vi "my_1D_sample-tip-convolution.vi"() -> ()   [LabVIEW 2017]
panel:
  out "Waveform Graph":dbl[][](graph)
  in  "stop":bool
  in  "scanning speed":u32(slide)=66 scale=1.0..1000.0
  in  "Angle":dbl=1.0 min=1.0 max=89.0 format="%.2f"
  in  "Radius":dbl min=-0.0 max=1000.0 format="%.2f"
  in  "Length":i32=1000
  in  "Period":dbl=310.0 format="%.2f"
  in  "Height":dbl=120.0 format="%.2f"
  in  "Width":dbl=140.0 format="%.2f"
  in  "Slope":dbl=1.0 format="%.2f"
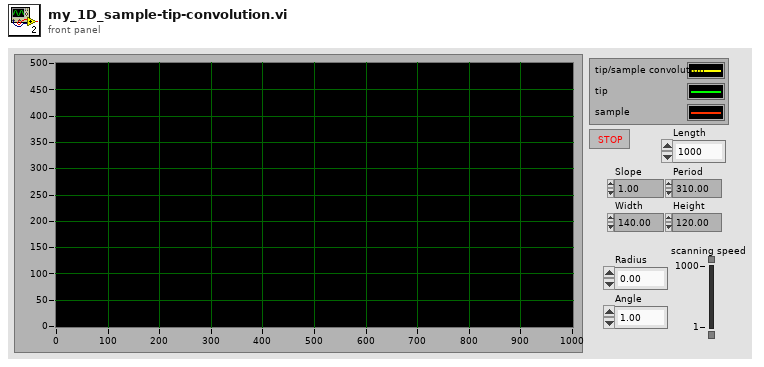
[diagram p1: front panel]
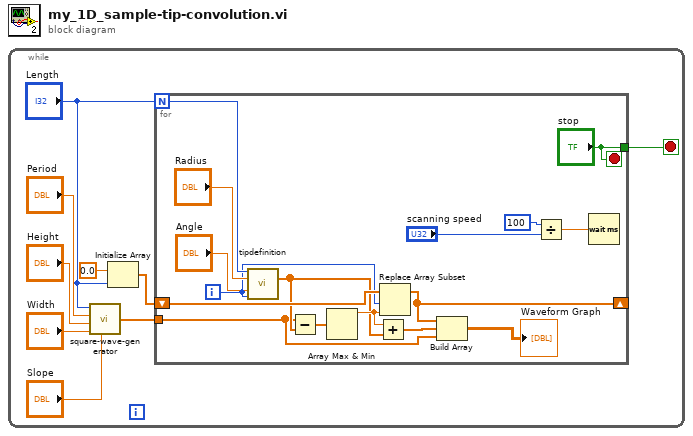
[diagram p0: block diagram]
diagram:
  n1 = while {
    stop <- w1 stop-if-true
    n2 = call "square-wave-generator.vi"("Slope"="Slope", "Width"="Width", "Height"="Height", "Period"="Period", "Length"="Length") -> ("Waveform Graph"=w5:dbl[])  [unwired: 1 in]
    n3 = Initialize Array(0.0 ("element"), "Length") -> (w2:dbl[])
    n4 = for {
      N: "Length" -> [w18]
      tunnel: w5 -> [w11]
      shift-right: [w13] -> _
      shift-left: w2 -> [w19]
      tunnel: ["stop"] -> w1
      i -> [w17]
      stop <- "stop" stop-if-true
      n5 = call "tipdefinition.vi"("#points"=w18, "radius of curvature"="Radius", "tipangle"="Angle", "offset"=w17) -> ("output"=w15:dbl[])  [unwired: 11 in]
      n6 = Subtract(x=w11, y=w15) -> (x-y=w20:dbl[])
      n7 = Array Max & Min(array=w20) -> (max value=w16:dbl)  [unwired: 3 out]
      n8 = Add(x=w16, y=w15) -> (x+y=w12:dbl[])
      n9 = Replace Array Subset(array=w19, new element=w16, index=w17) -> (w13:dbl[])
      n10 = Build Array(w13, w12, w11) -> (→"Waveform Graph":dbl[][])
      n11 = Divide(x=u32 100, y="scanning speed") -> (x/y=w23:dbl)
      n12 = Wait (ms)(milliseconds to wait=w23) -> ()  [unwired: 1 out]
    }
  }
